vi "Stanford Research SR1 Analog Generation.vi"() -> ()   [LabVIEW 2014]
doc: "This examples illustrates how to setup a new Analog Generator waveform and read its frequency out to a chart."
uses:
  Stanford Research SR1.lvlib
panel:
  in  "Stop Button":bool
  out "Frequency Chart":dbl(graph)
  in  "Type (0: awfSine)":i32(ring) items=["awfSine", "awfLoDistSine", "awfPhasedSine", "awfNoise", "awfUSASI", "awfSquare", "awfRamp", "awfArb", "awfChirp", "awfMultiTone", "awfIMD", "awfSyncBurstSine", "awfDC", "awfPolarity", "awfMLS", "awfLogSine"]
  in  "VISA resource name":refnum<visa-resource-name>
  # "(c) 2014 National Instruments.  ALL RIGHTS RESERVED."
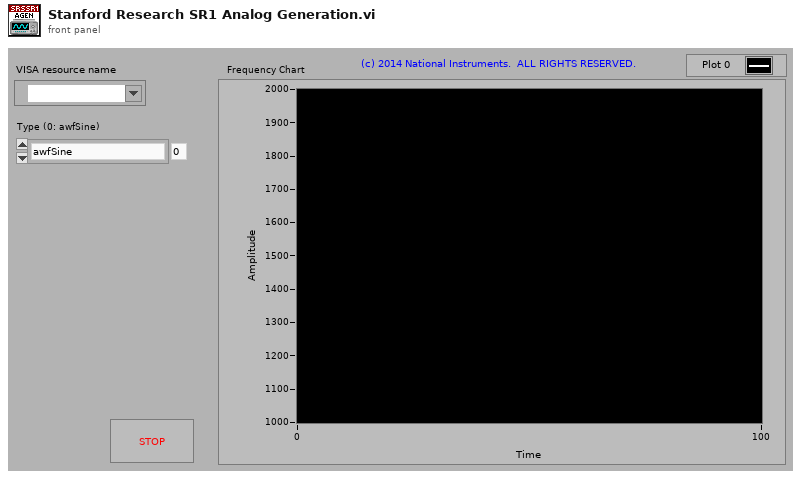
[diagram p1: front panel]
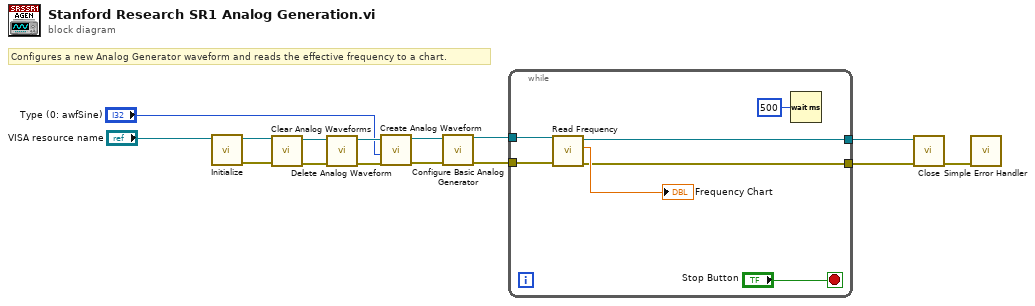
[diagram p0: block diagram]
diagram:
  # "Configures a new Analog Generator waveform and reads the effective frequency to a chart."
  n1 = call "Initialize.vi"("VISA resource name"="VISA resource name") -> ("error out"=w6:errorcluster, "VISA resource name out"=w7:refnum<visa-resource-name>)  [unwired: 9 in]
  n2 = call "Clear Analog Waveforms.vi"("error in (no error)"=w6, "VISA resource name"=w7) -> ("error out"=w4:errorcluster, "VISA resource name out"=w5:refnum<visa-resource-name>)  [unwired: 8 in]
  n3 = call "Delete Analog Waveform.vi"("error in (no error)"=w4, "VISA resource name"=w5) -> ("error out"=w2:errorcluster, "VISA resource name out"=w3:refnum<visa-resource-name>)  [unwired: 8 in]
  n4 = call "Create Analog Waveform.vi"("error in (no error)"=w2, "Type (0: awfSine)"="Type (0: awfSine)", "VISA resource name"=w3) -> ("error out"=w12:errorcluster, "VISA resource name out"=w13:refnum<visa-resource-name>)  [unwired: 6 in, 1 out]
  n5 = call "Configure Basic Analog Generator.vi"("VISA resource name"=w13, "error in (no error)"=w12) -> ("VISA resource name out"=w11:refnum<visa-resource-name>, "error out"=w10:errorcluster)  [unwired: 12 in]
  n6 = while {
    tunnel: w11 -> [w21]
    tunnel: w10 -> [w20]
    tunnel: [w18] -> w9
    tunnel: [w17] -> w8
    stop <- "Stop Button" stop-if-true
    n7 = call "Read Frequency.vi"("error in (no error)"=w20, "VISA resource name"=w21) -> ("error out"=w17:errorcluster, "Frequency"=→"Frequency Chart":dbl, "VISA resource name out"=w18:refnum<visa-resource-name>)  [unwired: 7 in]
    n8 = Wait (ms)(milliseconds to wait=u32 500) -> ()  [unwired: 1 out]
  }
  n9 = call "Close.vi"("error in (no error)"=w8, "VISA resource name"=w9) -> ("error out"=w14:errorcluster)  [unwired: 9 in]
  n10 = call <vilib>:"Simple Error Handler.vi"("error in (no error)"=w14) -> ()  [unwired: 4 in, 5 out]
